vi "JsonToCluster.vi"(8 "error in (no error)":errorcluster, 11 "Telemetry in":refnum<class "Telemetry.lvclass">) -> (0 "error out":errorcluster, 3 "Telemetry out":refnum<class "Telemetry.lvclass">)   [LabVIEW 2018, in "Telemetry.lvclass"]
uses:
  Telemetry.lvclass
  Telemetry.lvclass/Telemetry.ctl
panel:
  out "error JSON":errorcluster
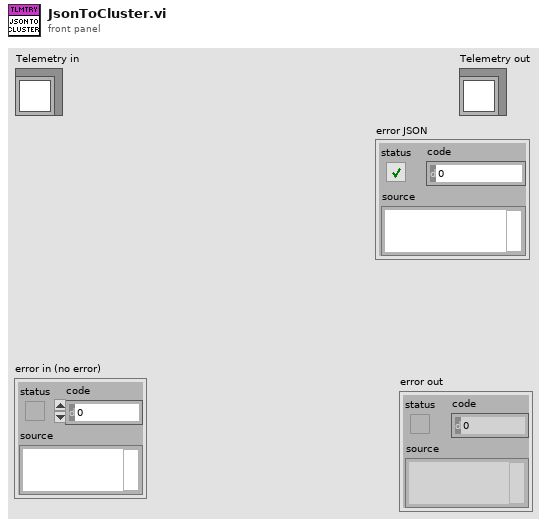
[diagram p1: front panel]
types:
  T1 = cluster{"broker":string, "version":string, "objectName":string, "raAcquis":string, "decAcquis":string, "epochAcquis":string, "airMass":string, "julianDate":string, "sideralTime":string, "hourAngle":string, "date":string, "time":string, "rightAscention":string, "declination":string, "guideStr":string, "guideAng":string, "guideNor":string, "guideEsp":string, "guideCas":string, "guidePlaca":string, "statShutter":string, "posCup":string, "raOnTarget":bool, "decOnTarget":bool, "dome":bool, "domeOnTarget":bool, "guider":bool, "mount":bool, "grossMovement":bool, "fineMovement":bool, "objCentrado":bool, "varTracking":bool, "shutter":bool, "cmd":string, "activeNST":string, "raNSTmove":string, "decNSTmove":string}
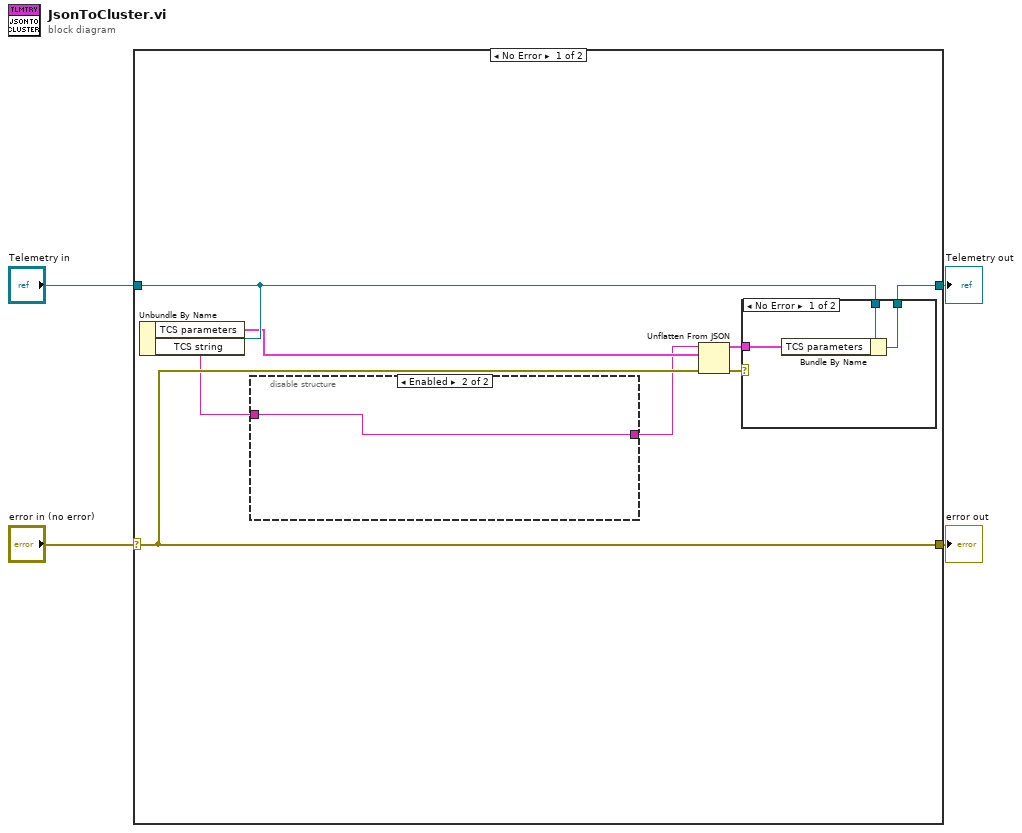
[diagram p0: block diagram]
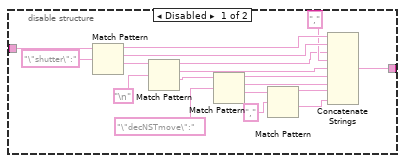
[diagram p2: hidden frame]
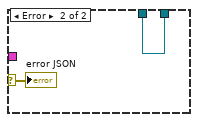
[diagram p3: hidden frame]
diagram:
  n1 = case shown="No Error" "error in (no error)" {
    selector: "error in (no error)" -> [w7 w38]
    tunnel: [w7 w38] -> w3
    tunnel: [w11 w37] -> w1
    tunnel: "Telemetry in" -> [w12 w37]
    frame No Error {
      n2 = Unbundle By Name(w12) -> ("TCS parameters"=w8:T1, "TCS string"=w6:string)
      n3 = disable-structure shown="Enabled" {
        disable-tunnel: w6 -> [w30 w31]
        disable-tunnel: [w26 w31] -> w5
        frame Disabled {
          n4 = Match Pattern(string=w30, regular expression="\"shutter\":") -> (before substring=w28:string, match substring=w27:string, after substring=w25:string)  [unwired: 1 in, 1 out]
          n5 = Match Pattern(string=w25, regular expression="\n") -> (before substring=w22:string, match substring=w21:string, after substring=w20:string)  [unwired: 1 in, 1 out]
          n6 = Match Pattern(string=w20, regular expression="\"decNSTmove\":") -> (before substring=w18:string, match substring=w17:string, after substring=w16:string)  [unwired: 1 in, 1 out]
          n7 = Match Pattern(string=w16, regular expression=",") -> (before substring=w14:string, after substring=w13:string)  [unwired: 1 in, 2 out]
          n8 = Concatenate Strings(w28, w27, w22, "," ("string"), w21, w18, w17, w14, w13) -> (w26:string)
        }
        frame Enabled {
        }
      }
      n9 = Unflatten From JSON(JSON string=w5, type and defaults=w8, error in (no error)=w7) -> (value=w10:T1, error out=w9:errorcluster)  [unwired: 4 in]
      n10 = case shown="No Error" w9 {
        selector: w9 -> [_ w36]
        tunnel: w12 -> [w34 w35]
        tunnel: [w33 w35] -> w11
        tunnel: w10 -> [w32 _]
        frame No Error {
          n11 = Bundle By Name(cluster=w34, "TCS parameters"=w32) -> (w33:refnum<class "Telemetry.lvclass">)
        }
        frame Error {
          "error JSON" <- w36
        }
      }
    }
    frame Error {
    }
  }
  "error out" <- w3
  "Telemetry out" <- w1
